vi "RigolRAP.vi"() -> ()   [LabVIEW 2009]
uses:
  <vilib>/Utility/file.llb/Write To Spreadsheet File (DBL).vi
panel:
  out "Histogram":waveform(i32)(graph)={"t0"=timestamp(22.5 s since 1904-01-01), "dt"=1.0, "Y"=[1, 1, 1, 1, 0, 6, 2, 2, 3, 4, 7, 6, 5, 10, 5, 12, 9, 9, 11, 8, 6, 6, 14, 4, 7, 2, 1, 3, 3, 3, 1, 0, 1, 0, 3, 0, 0, 0, 0, 0, 0, 0, 0, 0, 0, 0, 0, 0, 0, 0, 0, 0, 0, 0, 0, 0, 0, 0, 0, 0, 0, 0, 0, 0, 0, 0, 0, 0, 0, 0, 0, 0, 0, 0, 0, 0, 0, 0, 0, 0, 0, 0, 1, 0, 0, 0, 0, 1, 0, 0, 1, 0, 2, 0, 1, 2, 0, 2, 0, 4, 5, 0, 0, 2, 3, 2, 3, 8, 4, 7, 6, 3, 7, 5, 6, 9, 6, 8, 4, 10, 4, 4, 7, 7, 6, 8, 11, 7, 12, 6, 13, 6, 7, 12, 11, 11, 2, 4, 5, 6, 7, 5, 5, 4, 5, 4, 3, 2, 4, 6, 3, 2, 3, 1, 0, 4, 2, 1, 2, 1, 2, 1, 2, 2, 1, 1, 1, 1, 0, 0, 1, 1, 1, 0, 0, 2, 0, 0, 2]}
  out "Error":dbl
  out "Shelved Fraction":dbl
  in  "AP Sweep Width (MHz)":dbl
  in  "Sweep duration (ms)":dbl
  in  "RIGOL Vpp":dbl
  in  "1762 Frequency (MHz)":dbl=9.94 min=0.0 max=30000000.0
  in  "Comment":string="ARP it like it's hot"
  in  "B Field":dbl=0.85
  in  "Real Cutoff":dbl=20.0
  out "Shelving Events":dbl=11.0
  out "Dark Counts":dbl=19.0
  out "Bright Counts":dbl=61.0
  in  "Interval":dbl=0.02
  in  "OP Time (us)":dbl=3.0
  in  "Runs":dbl=40.0
  out "Path":path=path "c:/data/1762 Scans/2009-11-09_16-22-05_1762scanWithPumping.txt"
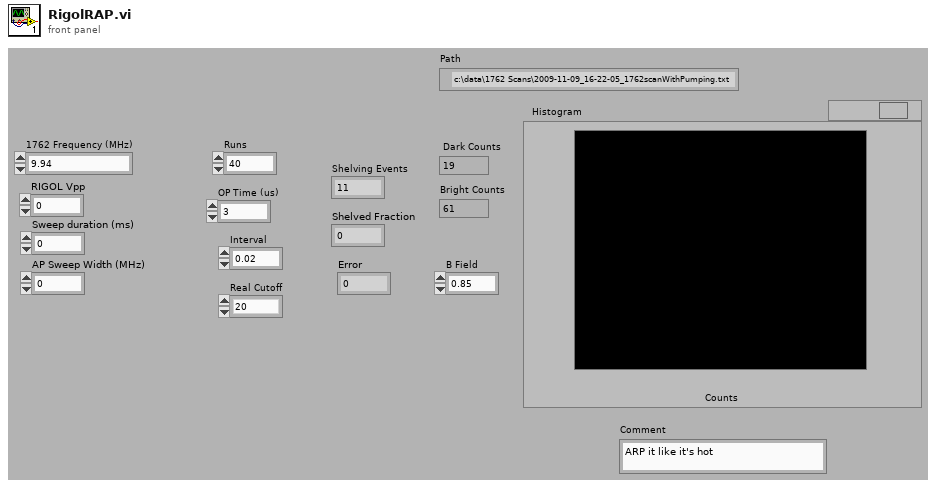
[diagram p1: front panel]
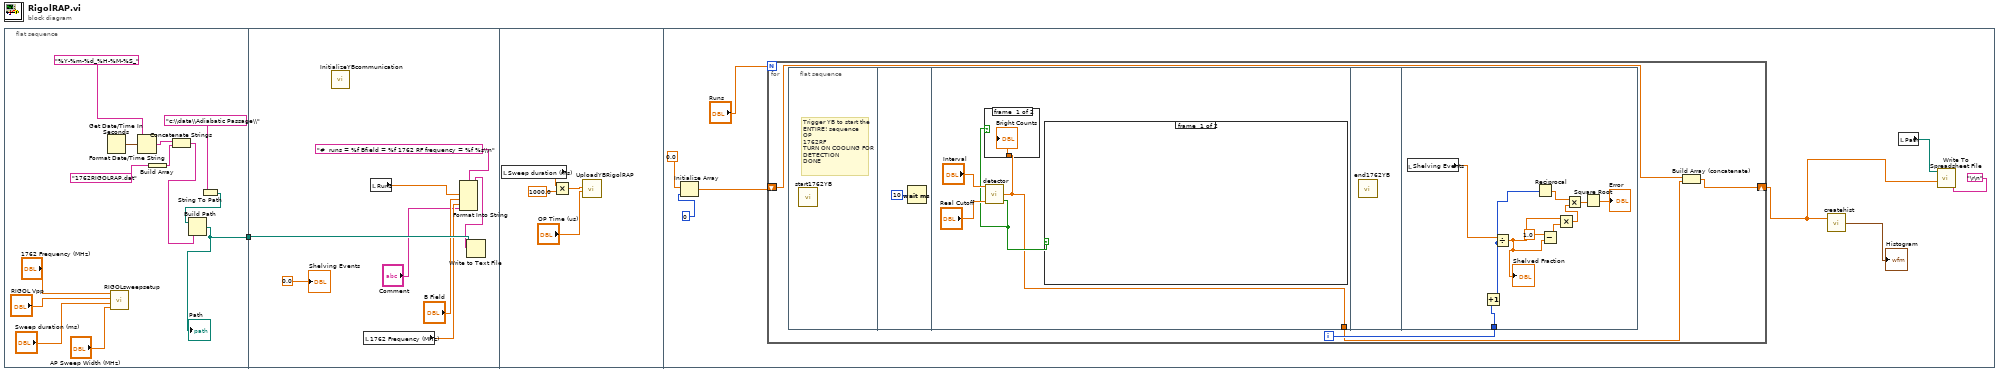
[diagram p0: block diagram]
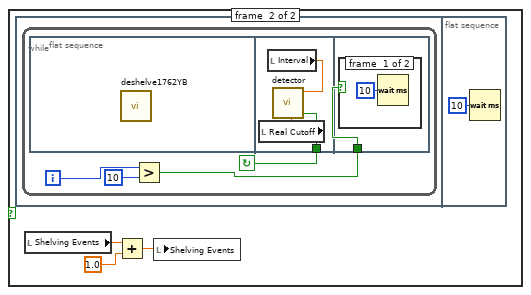
[diagram p2: hidden frame]
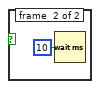
[diagram p3: hidden frame]
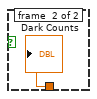
[diagram p4: hidden frame]
diagram:
  n1 = flat-sequence {
    tunnel: [w6] -> w1
    tunnel: w1 -> [w22]
    frame #0 {
      n2 = Get Date/Time In Seconds() -> (seconds since 1Jan1904=w8:timestamp)
      n3 = call "RIGOLsweepsetup.vi"("AP Sweep Width (MHz)"="AP Sweep Width (MHz)", "Time (ms)"="Sweep duration (ms)", "Amplitude (Vpp)"="RIGOL Vpp", "Frequency (MHz)"="1762 Frequency (MHz)") -> ()  [unwired: 8 in]
      n4 = Format Date/Time String(time format string (%c)="%Y-%m-%d_%H-%M-%S_", seconds (now)=w8) -> (date/time string=w10:string)  [unwired: 1 in]
      n5 = Build Array("1762RIGOLRAP.dat") -> (w13:string[])
      n6 = Concatenate Strings(w10, w13) -> (w12:string)
      n7 = String To Path(string="c:\\data\\Adiabatic Passage\\") -> (path=w14:path)
      n8 = Build Path(base path=w14, name or relative path=w12) -> (appended path=w6:path)
      "Path" <- w6
    }
    frame #1 {
      n9 = call "InitializeYBcommunication.vi"() -> ()  [unwired: 12 in]
      n10 = local read "1762 Frequency (MHz)"() -> (w17:dbl)
      n11 = local read "Runs"() -> (w19:dbl)
      n12 = Format Into String(format string="#  runs = %f Bfield = %f 1762 RF frequency = %f %s\\n", w19, "B Field", w17, "Comment") -> (resulting string=w20:string)  [unwired: 2 in, 1 out]
      n13 = Write to Text File(file (use dialog)=w22, text=w20) -> ()  [unwired: 2 in, 3 out]
      "Shelving Events" <- 0.0 ("Shelving Events")
    }
    frame #2 {
      n14 = local read "Sweep duration (ms)"() -> (w24:dbl)
      n15 = Multiply(x=w24, y=1000.0) -> (x*y=w25:dbl)
      n16 = call "UploadYBRigolRAP.vi"("OP Time"="OP Time (us)", "1762 Pulse Time"=w25) -> ()  [unwired: 10 in]
    }
    frame #3 {
      n17 = Initialize Array(0.0, 0) -> (w30:dbl[])
      n18 = for {
        N: "Runs" -> [_]
        shift-right: [w35] -> w29
        shift-left: w30 -> [w37]
        i -> [w38]
        n19 = flat-sequence {
          tunnel: [w40] -> w36
          tunnel: w38 -> [w63]
          frame #0 {
            # "Trigger YB to start the ENTIRE! sequence\nOP\n1762RF\nTURN ON COOLING FOR DETECTION\nDONE"
            n20 = call "start1762YB.vi"() -> ()  [unwired: 11 in, 1 out]
          }
          frame #1 {
            n21 = Wait (ms)(milliseconds to wait=u32 10) -> ()  [unwired: 1 out]
          }
          frame #2 {
            n22 = call "detector.vi"("Cutoff"="Real Cutoff", "Interval"="Interval") -> ("Boolean"=w41:bool, "Counts"=w40:dbl)  [unwired: 3 in]
            n23 = case shown="True" w41 {
              tunnel: w40 -> [w58 w59]
              frame #0 {
                "Bright Counts" <- w58
              }
              frame #1 {
                "Dark Counts" <- w59
              }
            }
            n24 = case shown="True" w41 {
              frame #0 {
              }
              frame #1 {
                n25 = flat-sequence {
                  frame #0 {
                    n26 = while {
                      i -> [w49]
                      stop <- w50 continue-if-true
                      n27 = flat-sequence {
                        tunnel: [w51] -> w50
                        tunnel: w47 -> [w54]
                        frame #0 {
                          n28 = call "deshelve1762YB.vi"() -> ()  [unwired: 11 in, 1 out]
                        }
                        frame #1 {
                          n29 = local read "Real Cutoff"() -> (w52:dbl)
                          n30 = local read "Interval"() -> (w53:dbl)
                          n31 = call "detector.vi"("Cutoff"=w52, "Interval"=w53) -> ("Boolean"=w51:bool)  [unwired: 3 in, 1 out]
                        }
                        frame #2 {
                          n32 = case shown="True" w54 {
                            frame #0 {
                              n33 = Wait (ms)(milliseconds to wait=u32 10) -> ()  [unwired: 1 out]
                            }
                            frame #1 {
                              n34 = Wait (ms)(milliseconds to wait=u32 10) -> ()  [unwired: 1 out]
                            }
                          }
                        }
                      }
                      n35 = Greater?(x=w49, y=10) -> (0:w47:bool)
                    }
                  }
                  frame #1 {
                    n36 = Wait (ms)(milliseconds to wait=u32 10) -> ()  [unwired: 1 out]
                  }
                }
                n37 = local read "Shelving Events"() -> (w45:dbl)
                n38 = Add(x=w45, y=1.0) -> (x+y=w44:dbl)
                n39 = local write "Shelving Events"(w44) -> ()
              }
            }
          }
          frame #3 {
            n40 = call "end1762YB.vi"() -> ()  [unwired: 1 in]
          }
          frame #4 {
            n41 = local read "Shelving Events"() -> (w64:dbl)
            n42 = Increment(x=w63) -> (x+1=w60:i32)
            n43 = Divide(x=w64, y=w60) -> (x/y=w62:dbl)
            "Shelved Fraction" <- w62
            n44 = Reciprocal(x=w60) -> (1/x=w69:dbl)
            n45 = Subtract(x=1.0, y=w62) -> (x-y=w67:dbl)
            n46 = Multiply(x=w62, y=w67) -> (x*y=w65:dbl)
            n47 = Multiply(x=w69, y=w65) -> (x*y=w68:dbl)
            n48 = Square Root(x=w68) -> (sqrt(x)=→"Error":dbl)
          }
        }
        n49 = Build Array (concatenate)(w37, w36) -> (w35:dbl[])
      }
      n50 = call "createhist.vi"("Array"=w29) -> ("Waveform Graph"=→"Histogram":waveform(i32))  [unwired: 1 in]
      n51 = local read "Path"() -> (w28:path)
      n52 = call-poly <vilib>:"Write To Spreadsheet File.vi"("delimiter (\\t)"="\r\n", "1D data"=w29, "file path (dialog if empty)"=w28) -> ()  [unwired: 5 in, 1 out]
    }
  }
